vi "HEWH Stand Overide.vi"() -> ()   [LabVIEW 2009]
uses:
  EquipReferences.ctl
  HEWH Tank Indicator.ctl
  Intellifaucet/Intellfaucet Mode.ctl
  PowerElements.ctl
  ChannelSettings.ctl
  <vilib>/Utility/file.llb/Write To Spreadsheet File (string).vi
panel:
  in  "Equipment":T1={"COM Port"="COM3", "MW100"="MW100", "AG34970"="A-34972A", "WT500"="WT500"}
  in  "Flow Calculation":bool
  out "Iteration":i32
  out "MW100":refnum<visa-resource-name>
  out "Local?":bool
  in  "Help":bool
  in  "VALVE OUT":enum8{"CLOSE", "OPEN"}(ring)
  in  "DRAIN VALVE":enum8{"OPEN", "CLOSE"}(ring)
  in  "INPUT VALVE":enum8{"OPEN", "CLOSE"}(ring)
  out "Error Out":errorcluster
  out "Ready":bool=TRUE
  in  "Stop Test":bool
  in  "HEWH Power":bool
  in  "Semiphore":T2
  in  "IF Stop":bool
  in  "IF Start":bool
  in  "IFaucet Driver":bool
  in  "Percent Flow":dbl(slide)=100.0 scale=0.0..100.0
  in  "Temperature(F)":dbl(slide)=58.0 scale=40.0..120.0
  in  "Mode":T3
  in  "Error In":errorcluster
  in  "Agilent?":bool=TRUE
  in  "No Serial Port Delay(mS, 250 mS increments)":u32=10000
  out "POWER":T4
  in  "Serial Port Available?":bool=TRUE
  in  "Write To File":bool
  in  "file path (dialog if empty)":path=path "C:/Data/data.csv"
  out "GatherDataCount":i32
  out "Output Data":string[][](array[string])
  out "Tank Display":T5 {"TC6" format="%.2g"; "TIN" format="%.2g"; "TOUT" format="%.2g"; "Mean" format="%.2f"; "Std Dev" format="%.2f"; "TC5" format="%.2g"; "TC4" format="%.2g"; "TC3" format="%.2g"; "TC2" format="%.2g"; "TC1" format="%.2g"}
  in  "Gather Data":bool
  in  "Test Condition":T6(ring)=enum."SRK500,Station1,5GPM FR"
  out "Dispensed":dbl
  out "ToutMin":dbl
  out "ToutMax":dbl
  in  "Gallon Target":dbl=10.72
  in  "GPM Target":dbl=3.0
  in  "Dispense":bool
  out "LBS":dbl
  in  "Reset Computations":bool
  out "Gallons":dbl
  out "BUG array":string[](array[string])
  out "Flow Chart":dbl(graph)
  out "Flow":dbl
  in  "Read Flow":bool
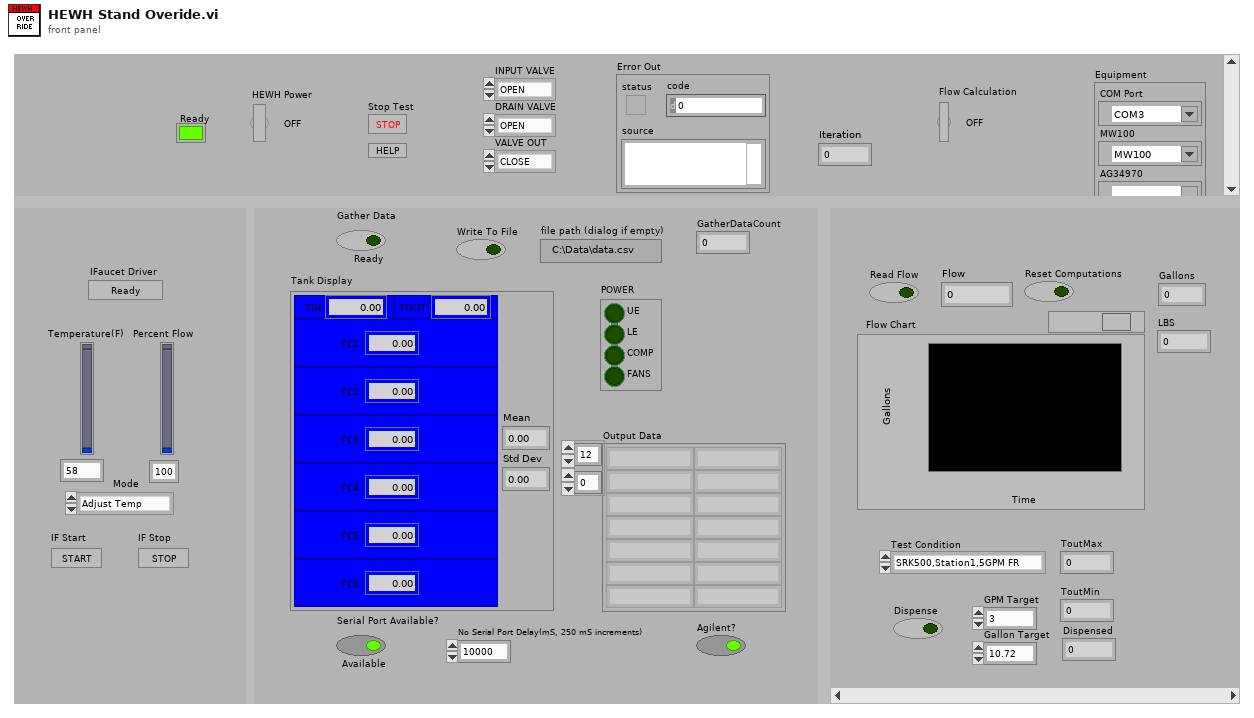
[diagram p1: front panel]
types:
  T1 = typedef "EquipReferences.ctl" = cluster{"COM Port":refnum<visa-resource-name>, "MW100":refnum<visa-resource-name>, "AG34970":refnum<visa-resource-name>, "WT500":refnum<visa-resource-name>}
  T2 = typedef "Semaphore RefNum" = refnum<k1>
  T3 = typedef "Intellfaucet Mode.ctl" = enum16{"Adjust Temp", "Adjust Flow", "Start Flow", "Stop Flow"}
  T4 = typedef "PowerElements.ctl" = cluster{"UE":bool, "LE":bool, "COMP":bool, "FANS":bool}
  T5 = typedef "HEWH Tank Indicator.ctl" = cluster{"TC1-D":bool, "TC2-D":bool, "TC3-D":bool, "TC4-D":bool, "TC5-D":bool, "RTD_IN":bool, "RTDOUT":bool, "TC1":dbl, "TC2":dbl, "TC3":dbl, "TC4":dbl, "TC5":dbl, "TIN":dbl, "TOUT":dbl, "Std Dev":dbl, "Mean":dbl, "TC6-D":bool, "TC6":dbl}
  T6 = enum16{"DRK500,Station1", "DRK375,Lab", "SRK500,Station1,5GPM FR", "DRK500,Station1,downspout"}
  T7 = typedef "ChannelSettings.ctl" = u32
  T8 = enum16{"Computation Start", "Computation stop", "Reset Computation", "Clear Computation"}
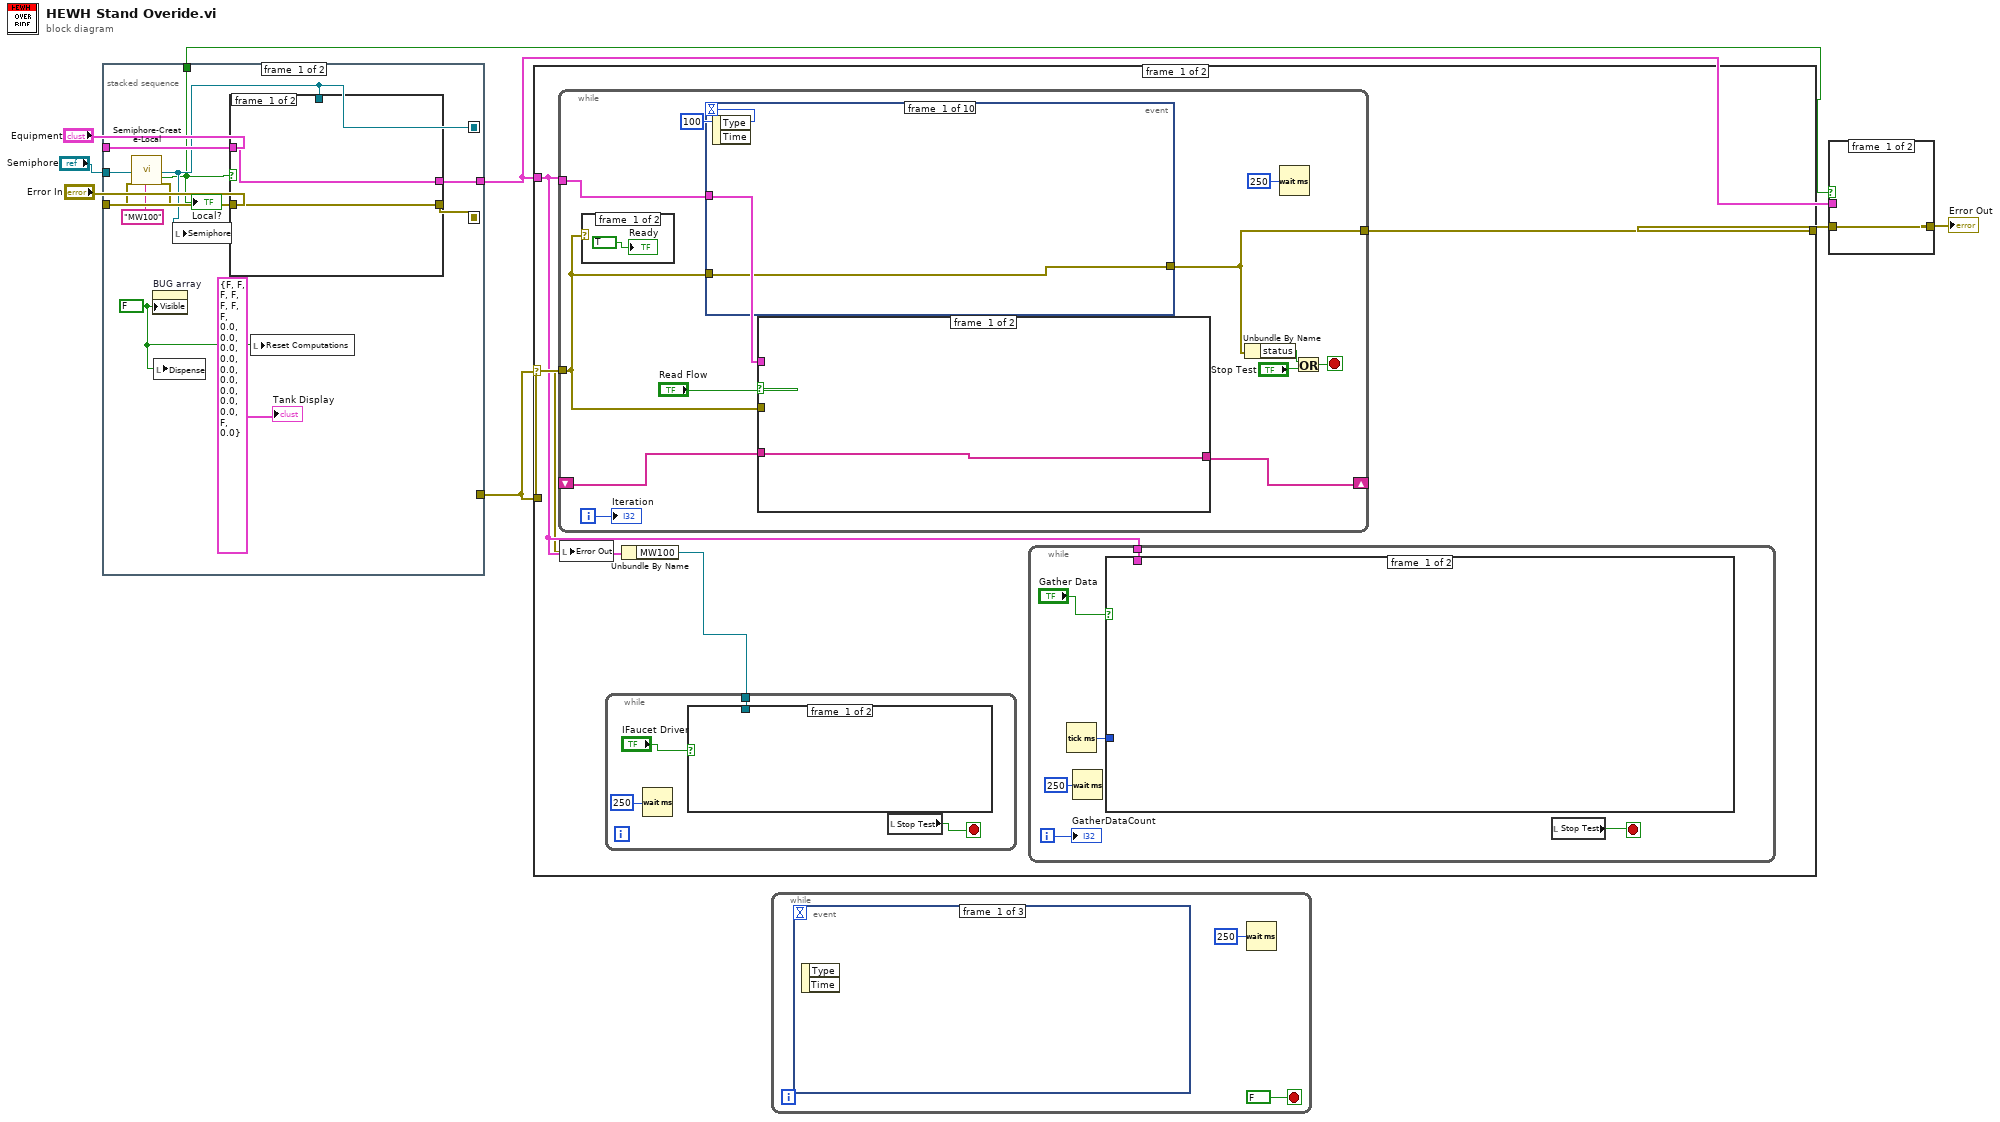
[diagram p0: block diagram]
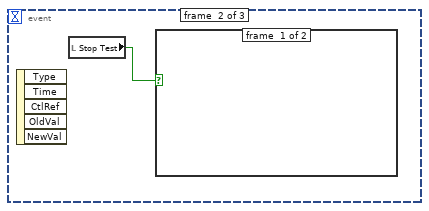
[diagram p2: hidden frame]
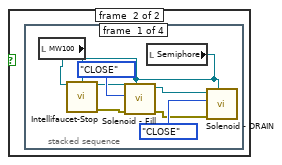
[diagram p3: hidden frame]
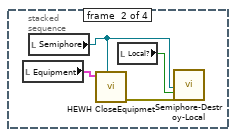
[diagram p4: hidden frame]
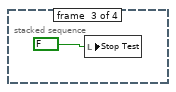
[diagram p5: hidden frame]
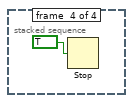
[diagram p6: hidden frame]
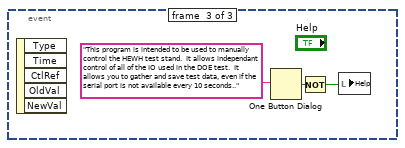
[diagram p7: hidden frame]
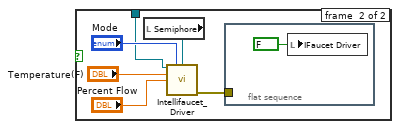
[diagram p8: hidden frame]
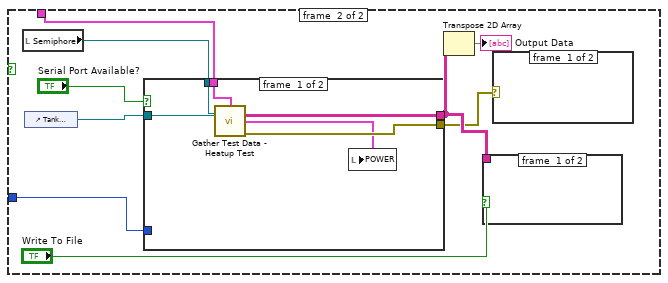
[diagram p9: hidden frame]
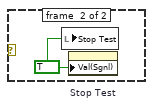
[diagram p10: hidden frame]
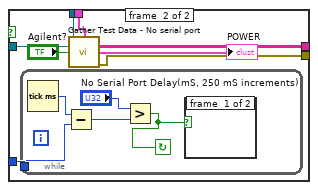
[diagram p11: hidden frame]
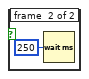
[diagram p12: hidden frame]
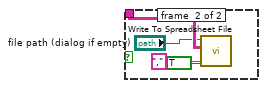
[diagram p13: hidden frame]
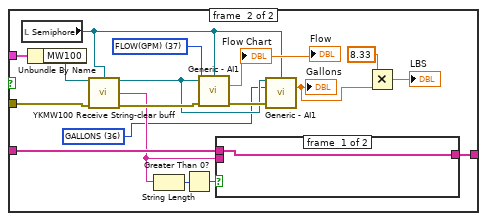
[diagram p14: hidden frame]
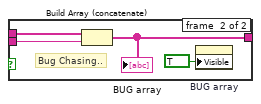
[diagram p15: hidden frame]
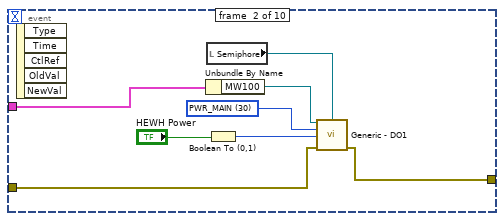
[diagram p17: hidden frame]
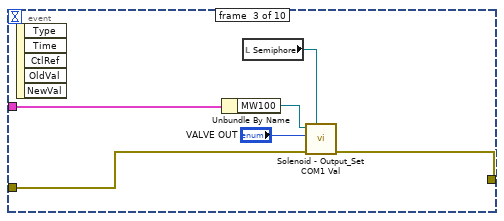
[diagram p18: hidden frame]
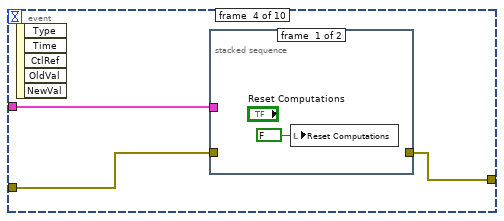
[diagram p19: hidden frame]
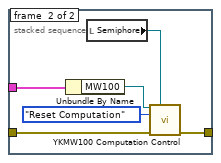
[diagram p20: hidden frame]
diagram:
  n1 = stacked-sequence {
    seq-local: [w17 _] -> [_ w45]
    seq-local: [w12 _] -> [_ w31]
    tunnel: "Error In" -> [w16 _]
    tunnel: "Equipment" -> [w19 w46]
    tunnel: [w18 _] -> w4
    tunnel: [_ w41] -> w3
    tunnel: [w11 _] -> w2
    tunnel: "Semiphore" -> [w14 _]
    frame #0 {
      w9 = FALSE ("Visible")
      n2 = call "Semiphore-Create-Local.vi"("Semiphore"=w14, "error in (no error)"=w16, "name (unnamed)"="MW100") -> ("semaphore"=w12:T2, "Local?"=w11:bool, "error out"=w15:errorcluster)  [unwired: 14 in]
      "Local?" <- w11
      n3 = property on="BUG array" class="Arr (strict)"("Visible"=w9) -> ()  [unwired: 2 in, 2 out]
      n4 = local write "Dispense"(w9) -> ()
      n5 = local write "Semiphore"(w12) -> ()
      n6 = case shown="True" w11 {
        tunnel: w15 -> [w21 w28]
        tunnel: [w21 w27] -> w17
        tunnel: w19 -> [w20 w26]
        tunnel: [w20 w23] -> w18
        tunnel: w12 -> [_ w24]
        frame #0 {
        }
        frame #1 {
          n7 = call "HEWH InitializeEquipmet.vi"("Semiphore"=w24, "Error In"=w28, "Equipment"=w26) -> ("Error Out"=w27:errorcluster, "Equipment Out"=w23:T1)  [unwired: 7 in]
          n8 = local write "Ready"(FALSE ("Ready")) -> ()
          n9 = Unbundle(w23) -> ("MW100"=→"MW100":refnum<visa-resource-name>)  [unwired: 3 out]
        }
      }
      n10 = local write "Reset Computations"(w9) -> ()
      "Tank Display" <- T5 {"TC1-D"=FALSE, "TC2-D"=FALSE, "TC3-D"=FALSE, "TC4-D"=FALSE, "TC5-D"=FALSE, "RTD_IN"=FALSE, "RTDOUT"=FALSE, "TC1"=0.0, "TC2"=0.0, "TC3"=0.0, "TC4"=0.0, "TC5"=0.0, "TIN"=0.0, "TOUT"=0.0, "Std Dev"=0.0, "Mean"=0.0, "TC6-D"=FALSE, "TC6"=0.0} ("Tank Display")
    }
    frame #1 {
      w32 = FALSE ("Stop Test")
      w36 = T7 30 items=["4-20_OUT", "Pres_HI1", "Pres_HI2", "Pres_LOW", "Pres_PIN", "HEATER_TOP", "HEATER_BOT", "T_Shell", "FLOWMETER", "WATT_SENSE", "WH_TICK", "Tc_1", "Tc_2", "Tc_3", "Tc_4", "Tc_5", "Tc_6", "Tc_down", "T_Shell_2", "T_Shell_3", "T_Shell_4", "RTD_IN", "RTD_OUT", "RTD_AMB", "INTF_TEMPFLO", "INTF_READY", "INTF_START", "INTF_STOP", "DRM_LOW", "DRM_HIGH", "PWR_MAIN", "VLV_DUMP", "VLV_OUT", "VLV_IN", "WATT_HOURS", "FLOW(SAMPLE)", "GALLONS", "FLOW(GPM)"] ("Channel_Enum")
      w37 = T7 33 items=["4-20_OUT", "Pres_HI1", "Pres_HI2", "Pres_LOW", "Pres_PIN", "HEATER_TOP", "HEATER_BOT", "T_Shell", "FLOWMETER", "WATT_SENSE", "WH_TICK", "Tc_1", "Tc_2", "Tc_3", "Tc_4", "Tc_5", "Tc_6", "Tc_down", "T_Shell_2", "T_Shell_3", "T_Shell_4", "RTD_IN", "RTD_OUT", "RTD_AMB", "INTF_TEMPFLO", "INTF_READY", "INTF_START", "INTF_STOP", "DRM_LOW", "DRM_HIGH", "PWR_MAIN", "VLV_DUMP", "VLV_OUT", "VLV_IN", "WATT_HOURS", "FLOW(SAMPLE)", "GALLONS", "FLOW(GPM)"] ("Channel_Enum")
      w38 = T7 32 items=["4-20_OUT", "Pres_HI1", "Pres_HI2", "Pres_LOW", "Pres_PIN", "HEATER_TOP", "HEATER_BOT", "T_Shell", "FLOWMETER", "WATT_SENSE", "WH_TICK", "Tc_1", "Tc_2", "Tc_3", "Tc_4", "Tc_5", "Tc_6", "Tc_down", "T_Shell_2", "T_Shell_3", "T_Shell_4", "RTD_IN", "RTD_OUT", "RTD_AMB", "INTF_TEMPFLO", "INTF_READY", "INTF_START", "INTF_STOP", "DRM_LOW", "DRM_HIGH", "PWR_MAIN", "VLV_DUMP", "VLV_OUT", "VLV_IN", "WATT_HOURS", "FLOW(SAMPLE)", "GALLONS", "FLOW(GPM)"] ("Channel_Enum")
      w40 = T7 31 items=["4-20_OUT", "Pres_HI1", "Pres_HI2", "Pres_LOW", "Pres_PIN", "HEATER_TOP", "HEATER_BOT", "T_Shell", "FLOWMETER", "WATT_SENSE", "WH_TICK", "Tc_1", "Tc_2", "Tc_3", "Tc_4", "Tc_5", "Tc_6", "Tc_down", "T_Shell_2", "T_Shell_3", "T_Shell_4", "RTD_IN", "RTD_OUT", "RTD_AMB", "INTF_TEMPFLO", "INTF_READY", "INTF_START", "INTF_STOP", "DRM_LOW", "DRM_HIGH", "PWR_MAIN", "VLV_DUMP", "VLV_OUT", "VLV_IN", "WATT_HOURS", "FLOW(SAMPLE)", "GALLONS", "FLOW(GPM)"] ("Channel_Enum")
      n11 = Unbundle By Name(w46) -> ("MW100"=w39:refnum<visa-resource-name>)
      n12 = local write "Stop Test"(w32) -> ()
      n13 = local write "Ready"(w32) -> ()
      n14 = local write "IFaucet Driver"(w32) -> ()
      n15 = call "YKMW100 VF0 Relay Status.vi"("VISA session"=w39, "Semiphore"=w31, "Channel_Enum"=w36, "error in (no error)"=w45) -> ("x = y?"=w29:bool, "error out"=w44:errorcluster)  [unwired: 9 in, 1 out]
      n16 = call "YKMW100 VF0 Relay Status.vi"("VISA session"=w39, "Semiphore"=w31, "Channel_Enum"=w37, "error in (no error)"=w44) -> ("x = y?"=w35:bool, "error out"=w43:errorcluster)  [unwired: 9 in, 1 out]
      n17 = call "YKMW100 VF0 Relay Status.vi"("VISA session"=w39, "Semiphore"=w31, "Channel_Enum"=w38, "error in (no error)"=w43) -> ("x = y?"=w34:bool, "error out"=w42:errorcluster)  [unwired: 9 in, 1 out]
      n18 = call "YKMW100 VF0 Relay Status.vi"("VISA session"=w39, "Semiphore"=w31, "Channel_Enum"=w40, "error in (no error)"=w42) -> ("x = y?"=w33:bool, "error out"=w41:errorcluster)  [unwired: 9 in, 1 out]
      n19 = Not(x=w29) -> (.not. x?=w30:bool)
      n20 = case shown="False" w35 {
        frame #0 {
          n21 = local write "INPUT VALVE"(enum8{"OPEN", "CLOSE"}."CLOSE" ("INPUT VALVE")) -> ()
        }
        frame #1 {
          n22 = local write "INPUT VALVE"(enum8{"OPEN", "CLOSE"}."OPEN" ("INPUT VALVE")) -> ()
        }
      }
      n23 = case shown="False" w33 {
        frame #0 {
          n24 = local write "DRAIN VALVE"(enum8{"OPEN", "CLOSE"}."OPEN" ("DRAIN VALVE")) -> ()
        }
        frame #1 {
          n25 = local write "DRAIN VALVE"(enum8{"OPEN", "CLOSE"}."CLOSE" ("DRAIN VALVE")) -> ()
        }
      }
      n26 = case shown="False" w34 {
        frame #0 {
          n27 = local write "VALVE OUT"(enum8{"CLOSE", "OPEN"}."CLOSE" ("VALVE OUT")) -> ()
        }
        frame #1 {
          n28 = local write "VALVE OUT"(enum8{"CLOSE", "OPEN"}."OPEN" ("VALVE OUT")) -> ()
        }
      }
      n29 = local write "HEWH Power"(w30) -> ()
    }
  }
  n30 = case shown="No Error" w3 {
    selector: w3 -> [w53 _]
    tunnel: [w57 w216] -> w7
    tunnel: w3 -> [w56 w216]
    tunnel: w4 -> [w55 _]
    frame #0 {
      n31 = while {
        tunnel: w56 -> [w111]
        tunnel: [w116] -> w57
        shift-right: [w113] -> _
        shift-left: _ -> [w112]
        tunnel: w55 -> [w110]
        i -> [w114]
        stop <- w117 stop-if-true
        n32 = case shown="No Error" w111 {
          frame #0 {
            "Ready" <- TRUE
          }
          frame #1 {
          }
        }
        n33 = event shown="[7] \"IF Start\": Value Change" {
          selector: _ -> [_ _ _ _ _ _ _ _ _ _]
          dyn-events: _ -> [_ _ _ _ _ _ _ _ _ _]
          timeout: 100 -> [_ _ _ _ _ _ _ _ _ _]
          tunnel: w111 -> [w146 w152 w156 w162 w181 w186 w190 w196 w203 w211]
          tunnel: [w146 w148 w157 w161 w173 w185 w189 w195 w202 w210] -> w116
          tunnel: w110 -> [_ w151 w160 w163 w180 w188 w194 w199 w205 w214]
          event #0 {
            n34 = event-data() -> ()  [unwired: 1 in, 2 out]
          }
          event #1 {
            w150 = T7 30 items=["4-20_OUT", "Pres_HI1", "Pres_HI2", "Pres_LOW", "Pres_PIN", "HEATER_TOP", "HEATER_BOT", "T_Shell", "FLOWMETER", "WATT_SENSE", "WH_TICK", "Tc_1", "Tc_2", "Tc_3", "Tc_4", "Tc_5", "Tc_6", "Tc_down", "T_Shell_2", "T_Shell_3", "T_Shell_4", "RTD_IN", "RTD_OUT", "RTD_AMB", "INTF_TEMPFLO", "INTF_READY", "INTF_START", "INTF_STOP", "DRM_LOW", "DRM_HIGH", "PWR_MAIN", "VLV_DUMP", "VLV_OUT", "VLV_IN", "WATT_HOURS", "FLOW(SAMPLE)", "GALLONS", "FLOW(GPM)"] ("Channel_Enum")
            n35 = event-data() -> ()  [unwired: 1 in, 5 out]
            n36 = Unbundle By Name(w151) -> ("MW100"=w153:refnum<visa-resource-name>)
            n37 = local read "Semiphore"() -> (w149:T2)
            n38 = Boolean To (0,1)(Boolean="HEWH Power") -> (0, 1=w154:i16)
            n39 = call "Generic - DO1.vi"("VISA session"=w153, "Semiphore"=w149, "Channel_Enum"=w150, "Relay Status (0:CLOSED)"=w154, "Error In"=w152) -> ("error out"=w148:errorcluster)  [unwired: 9 in, 1 out]
          }
          event #2 {
            n40 = event-data() -> ()  [unwired: 1 in, 5 out]
            n41 = Unbundle By Name(w160) -> ("MW100"=w159:refnum<visa-resource-name>)
            n42 = local read "Semiphore"() -> (w158:T2)
            n43 = call "Solenoid - Output_Set COM1 Val.vi"("Semiphore"=w158, "Error In"=w156, "OPEN CLOSE"="VALVE OUT", "VISA session"=w159) -> ("Error Out"=w157:errorcluster)  [unwired: 6 in, 1 out]
          }
          event #3 {
            n44 = event-data() -> ()  [unwired: 1 in, 5 out]
            n45 = stacked-sequence {
              tunnel: w163 -> [_ w170]
              tunnel: w162 -> [_ w167]
              tunnel: [_ w165] -> w161
              frame #0 {
                n46 = local write "Reset Computations"(FALSE ("Reset Computations")) -> ()
              }
              frame #1 {
                n47 = Unbundle By Name(w170) -> ("MW100"=w169:refnum<visa-resource-name>)
                n48 = local read "Semiphore"() -> (w168:T2)
                n49 = call "YKMW100 Computation Control.vi"("VISA session"=w169, "Semiphore"=w168, "Mode"=T8."Reset Computation", "error in (no error)"=w167) -> ("error out"=w165:errorcluster)  [unwired: 10 in, 1 out]
              }
            }
          }
          event #4 {
            n50 = event-data() -> ()  [unwired: 1 in, 5 out]
            n51 = control-ref of="Flow Chart"() -> (w172:refnum<vi>)
            n52 = local read "Semiphore"() -> (w179:T2)
            n53 = call "Dispense X Gallon at Y Flowrate.vi"("Gallon Target"="Gallon Target", "Equipment"=w180, "Semiphore"=w179, "GPM Target"="GPM Target", "Test Condition"="Test Condition", "Error In"=w181, "Ctl Refnum"=w172) -> ("M*(Gallons)"=→"Dispensed":dbl, "ToutMax"=→"ToutMax":dbl, "ToutMin"=→"ToutMin":dbl, "Error Out"=w173:errorcluster)  [unwired: 3 in, 2 out]
            n54 = flat-sequence {
              tunnel: w173 -> [_]
              frame #0 {
                n55 = local write "Dispense"(FALSE ("IF Start")) -> ()
              }
            }
          }
          event #5 {
            n56 = event-data() -> ()  [unwired: 1 in, 5 out]
            n57 = Unbundle By Name(w188) -> ("MW100"=w183:refnum<visa-resource-name>)
            n58 = local read "Semiphore"() -> (w184:T2)
            n59 = call "Solenoid - Fill.vi"("Semiphore"=w184, "Error In"=w186, "VALVE OPEN CLOSE"="INPUT VALVE", "VISA session"=w183) -> ("Error Out"=w185:errorcluster)  [unwired: 6 in, 1 out]
          }
          event #6 {
            n60 = event-data() -> ()  [unwired: 1 in, 5 out]
            n61 = Unbundle By Name(w194) -> ("MW100"=w192:refnum<visa-resource-name>)
            n62 = local read "Semiphore"() -> (w193:T2)
            n63 = call "Solenoid - DRAIN.vi"("Semiphore"=w193, "Error In"=w190, "VALVE OPEN CLOSE"="DRAIN VALVE", "VISA session"=w192) -> ("Error Out"=w189:errorcluster)  [unwired: 6 in, 1 out]
          }
          event #7 {
            n64 = event-data() -> ()  [unwired: 1 in, 5 out]
            n65 = Unbundle By Name(w199) -> ("MW100"=w197:refnum<visa-resource-name>)
            n66 = local read "Semiphore"() -> (w198:T2)
            n67 = call "Intellifaucet-Start.vi"("Semiphore"=w198, "Error In"=w196, "VISA session"=w197) -> ("Error Out"=w195:errorcluster)  [unwired: 7 in, 1 out]
            n68 = flat-sequence {
              tunnel: w195 -> [_]
              frame #0 {
                n69 = local write "IF Start"(FALSE ("IF Start")) -> ()
              }
            }
          }
          event #8 {
            n70 = event-data() -> ()  [unwired: 1 in, 5 out]
            n71 = Unbundle By Name(w205) -> ("MW100"=w204:refnum<visa-resource-name>)
            n72 = local read "Semiphore"() -> (w201:T2)
            n73 = Select(t="001" ("Value"), s="Flow Calculation", f="000" ("Value")) -> (s? t:f=w206:string)
            n74 = call "YKMW100 Write Com Register.vi"("VISA session"=w204, "Semiphore"=w201, "Value"=w206, "error in (no error)"=w203) -> ("error out"=w202:errorcluster)  [unwired: 10 in, 1 out]
          }
          event #9 {
            n75 = event-data() -> ()  [unwired: 1 in, 5 out]
            n76 = Unbundle By Name(w214) -> ("MW100"=w212:refnum<visa-resource-name>)
            n77 = local read "Semiphore"() -> (w213:T2)
            n78 = call "Intellifaucet-Stop.vi"("VISA session"=w212, "Semiphore"=w213, "Error In"=w211) -> ("Error Out"=w210:errorcluster)  [unwired: 11 in, 1 out]
            n79 = flat-sequence {
              tunnel: w210 -> [_]
              frame #0 {
                n80 = local write "IF Stop"(FALSE ("IF Start")) -> ()
              }
            }
          }
        }
        n81 = case shown="True" "Read Flow" {
          tunnel: w110 -> [_ w139]
          tunnel: w111 -> [_ w137]
          tunnel: [w121 w135] -> w113
          tunnel: w112 -> [w121 w134]
          frame #0 {
          }
          frame #1 {
            w125 = T7 36 items=["4-20_OUT", "Pres_HI1", "Pres_HI2", "Pres_LOW", "Pres_PIN", "HEATER_TOP", "HEATER_BOT", "T_Shell", "FLOWMETER", "WATT_SENSE", "WH_TICK", "Tc_1", "Tc_2", "Tc_3", "Tc_4", "Tc_5", "Tc_6", "Tc_down", "T_Shell_2", "T_Shell_3", "T_Shell_4", "RTD_IN", "RTD_OUT", "RTD_AMB", "INTF_TEMPFLO", "INTF_READY", "INTF_START", "INTF_STOP", "DRM_LOW", "DRM_HIGH", "PWR_MAIN", "VLV_DUMP", "VLV_OUT", "VLV_IN", "WATT_HOURS", "FLOW(SAMPLE)", "GALLONS", "FLOW(GPM)"] ("Channel_Enum")
            w130 = T7 37 items=["4-20_OUT", "Pres_HI1", "Pres_HI2", "Pres_LOW", "Pres_PIN", "HEATER_TOP", "HEATER_BOT", "T_Shell", "FLOWMETER", "WATT_SENSE", "WH_TICK", "Tc_1", "Tc_2", "Tc_3", "Tc_4", "Tc_5", "Tc_6", "Tc_down", "T_Shell_2", "T_Shell_3", "T_Shell_4", "RTD_IN", "RTD_OUT", "RTD_AMB", "INTF_TEMPFLO", "INTF_READY", "INTF_START", "INTF_STOP", "DRM_LOW", "DRM_HIGH", "PWR_MAIN", "VLV_DUMP", "VLV_OUT", "VLV_IN", "WATT_HOURS", "FLOW(SAMPLE)", "GALLONS", "FLOW(GPM)"] ("Channel_Enum")
            n82 = local read "Semiphore"() -> (w126:T2)
            n83 = Unbundle By Name(w139) -> ("MW100"=w138:refnum<visa-resource-name>)
            n84 = call "YKMW100 Receive String-clear buff.vi"("VISA session"=w138, "Semiphore"=w126, "error in (no error)"=w137) -> ("dup VISA session"=w127:refnum<visa-resource-name>, "Read Buffer"=w133:string, "error out"=w136:errorcluster)  [unwired: 10 in]
            n85 = String Length(string=w133) -> (length=w132:i32)
            n86 = Greater Than 0?(x=w132) -> (x > 0?=w131:bool)
            n87 = call "Generic - AI1.vi"("MW100"=w127, "Semiphore"=w126, "Channel_Enum"=w130, "Error In"=w136) -> ("Value"=→"Flow" →"Flow Chart":dbl, "Error Out"=w128:errorcluster)  [unwired: 9 in, 1 out]
            n88 = case shown="True" w131 {
              tunnel: w133 -> [_ w144]
              tunnel: [w140 w142] -> w135
              tunnel: w134 -> [w140 w143]
              frame #0 {
              }
              frame #1 {
                # "Bug Chasing.."
                n89 = Build Array (concatenate)(w143, w144) -> (w142:string[])
                "BUG array" <- w142
                n90 = property on="BUG array" class="Arr (strict)"("Visible"=TRUE) -> ()  [unwired: 2 in, 2 out]
              }
            }
            n91 = call "Generic - AI1.vi"("MW100"=w127, "Semiphore"=w126, "Channel_Enum"=w125, "Error In"=w128) -> ("Value"=w124:dbl)  [unwired: 9 in, 2 out]
            "Gallons" <- w124
            n92 = Multiply(x=8.33, y=w124) -> (x*y=→"LBS":dbl)
          }
        }
        n93 = Unbundle By Name(w116) -> ("status"=w118:bool)
        n94 = Wait (ms)(milliseconds to wait=u32 250) -> ()  [unwired: 1 out]
        n95 = Or(x=w118, y="Stop Test") -> (x .or. y?=w117:bool)
        "Iteration" <- w114
      }
      n96 = local write "Error Out"(w53) -> ()
      n97 = Unbundle By Name(w55) -> ("MW100"=w54:refnum<visa-resource-name>)
      n98 = while {
        tunnel: w54 -> [w59]
        stop <- w60 stop-if-true
        n99 = Wait (ms)(milliseconds to wait=u32 250) -> ()  [unwired: 1 out]
        n100 = case shown="True" "IFaucet Driver" {
          tunnel: w59 -> [_ w63]
          frame #0 {
          }
          frame #1 {
            n101 = local read "Semiphore"() -> (w67:T2)
            n102 = call "Intellifaucet_Driver.vi"("VISA session"=w63, "Mode"="Mode", "Semiphore"=w67, "Temperature(F)"="Temperature(F)", "Percent Flow"="Percent Flow") -> ("Error Out"=w62:errorcluster)  [unwired: 9 in, 1 out]
            n103 = flat-sequence {
              tunnel: w62 -> [_]
              frame #0 {
                n104 = local write "IFaucet Driver"(FALSE ("IFaucet Driver")) -> ()
              }
            }
          }
        }
        n105 = local read "Stop Test"() -> (w60:bool)
      }
      n106 = while {
        tunnel: w55 -> [w72]
        i -> [w71]
        stop <- w73 stop-if-true
        n107 = Tick Count (ms)() -> (millisecond timer value=w69:u32)
        n108 = Wait (ms)(milliseconds to wait=u32 250) -> ()  [unwired: 1 out]
        n109 = case shown="True" "Gather Data" {
          tunnel: w72 -> [_ w80]
          tunnel: w69 -> [_ w75]
          frame #0 {
          }
          frame #1 {
            n110 = local read "Semiphore"() -> (w82:T2)
            n111 = control-ref of="Tank Display"() -> (w81:refnum<vi>)
            n112 = case shown="False" "Serial Port Available?" {
              tunnel: w82 -> [w90 w98]
              tunnel: w81 -> [w89 w97]
              tunnel: w80 -> [w88 w96]
              tunnel: [w87 w95] -> w79
              tunnel: [w86 w94] -> w76
              tunnel: w75 -> [_ w92]
              frame #0 {
                n113 = call "Gather Test Data - Heatup Test.vi"("Semiphore"=w90, "Equipment"=w88, "Tank Display Ref"=w89) -> ("Output Data"=w87:string[][], "POWER"=w85:T4, "error out"=w86:errorcluster)  [unwired: 8 in, 2 out]
                n114 = local write "POWER"(w85) -> ()
              }
              frame #1 {
                n115 = while {
                  tunnel: w92 -> [w102]
                  stop <- w99 continue-if-true
                  n116 = Tick Count (ms)() -> (millisecond timer value=w103:u32)
                  n117 = Subtract(x=w103, y=w102) -> (x-y=w100:u32)
                  n118 = Greater?(x="No Serial Port Delay(mS, 250 mS increments)", y=w100) -> (0:w99:bool)
                  n119 = case shown="True" w99 {
                    frame #0 {
                    }
                    frame #1 {
                      n120 = Wait (ms)(milliseconds to wait=u32 250) -> ()  [unwired: 1 out]
                    }
                  }
                }
                n121 = call "Gather Test Data - No serial port.vi"("Semiphore"=w98, "Equipment"=w96, "Tank Display Ref"=w97, "Agilent?"="Agilent?") -> ("Output Data"=w95:string[][], "POWER"=→"POWER":T4, "error out"=w94:errorcluster)  [unwired: 7 in, 2 out]
              }
            }
            n122 = Transpose 2D Array(2D array=w79) -> (transposed array=→"Output Data":string[][])
            n123 = case shown="True" "Write To File" {
              tunnel: w79 -> [_ w108]
              frame #0 {
              }
              frame #1 {
                n124 = call-poly <vilib>:"Write To Spreadsheet File.vi"("delimiter (\\t)"="," ("delimiter (\\t)"), "append to file? (new file:F)"=TRUE, "2D data"=w108, "file path (dialog if empty)"="file path (dialog if empty)") -> ()  [unwired: 4 in, 1 out]
              }
            }
            n125 = case shown="Error" w76 {
              frame #0 {
              }
              frame #1 {
                w84 = TRUE ("Value (Signaling)")
                n126 = local write "Stop Test"(w84) -> ()
                n127 = property on="Stop Test" class="Bool (strict)"("Val(Sgnl)"=w84) -> ()  [unwired: 2 in, 2 out]
              }
            }
          }
        }
        n128 = local read "Stop Test"() -> (w73:bool)
        "GatherDataCount" <- w71
      }
    }
    frame #1 {
    }
  }
  n129 = while {
    stop <- FALSE stop-if-true
    n130 = event shown="[1] \"Stop Test\": Value Change" {
      selector: _ -> [_ _ _]
      dyn-events: _ -> [_ _ _]
      timeout: _ -> [_ _ _]
      event #0 {
        n131 = event-data() -> ()  [unwired: 1 in, 2 out]
      }
      event #1 {
        n132 = event-data() -> ()  [unwired: 1 in, 5 out]
        n133 = local read "Stop Test"() -> (w219:bool)
        n134 = case shown="True" w219 {
          frame #0 {
          }
          frame #1 {
            n135 = stacked-sequence {
              frame #0 {
                n136 = local read "MW100"() -> (w221:refnum<visa-resource-name>)
                n137 = local read "Semiphore"() -> (w220:T2)
                n138 = call "Intellifaucet-Stop.vi"("VISA session"=w221, "Semiphore"=w220) -> ("dup VISA session"=w223:refnum<visa-resource-name>, "Error Out"=w227:errorcluster)  [unwired: 12 in]
                n139 = call "Solenoid - Fill.vi"("Semiphore"=w220, "Error In"=w227, "VALVE OPEN CLOSE"=enum8{"OPEN", "CLOSE"}."CLOSE", "VISA session"=w223) -> ("Error Out"=w225:errorcluster, "dup VISA session"=w222:refnum<visa-resource-name>)  [unwired: 6 in]
                n140 = call "Solenoid - DRAIN.vi"("Semiphore"=w220, "Error In"=w225, "VALVE OPEN CLOSE"=enum8{"OPEN", "CLOSE"}."CLOSE", "VISA session"=w222) -> ()  [unwired: 6 in, 2 out]
              }
              frame #1 {
                n141 = local read "Equipment"() -> (w231:T1)
                n142 = local read "Semiphore"() -> (w230:T2)
                n143 = call "HEWH CloseEquipmet.vi"("Semiphore"=w230, "Equipment"=w231) -> ("Error Out"=w229:errorcluster)  [unwired: 9 in]
                n144 = local read "Local?"() -> (w228:bool)
                n145 = call "Semiphore-Destroy-Local.vi"("Semiphore"=w230, "Local?"=w228, "error in (no error)"=w229) -> ()  [unwired: 16 in, 1 out]
              }
              frame #2 {
                n146 = local write "Stop Test"(FALSE ("stop")) -> ()
              }
              frame #3 {
                n147 = Stop(stop? (T)=TRUE) -> ()
              }
            }
          }
        }
      }
      event #2 {
        n148 = event-data() -> ()  [unwired: 1 in, 5 out]
        n149 = One Button Dialog(message="This program is intended to be used to manually control the HEWH test stand.  It allows independant control of all of the IO used in the DOE test.  It allows you to gather and save test data, even if the serial port is not available every 10 seconds..") -> (true=w235:bool)  [unwired: 1 in]
        n150 = Not(x=w235) -> (.not. x?=w234:bool)
        n151 = local write "Help"(w234) -> ()
      }
    }
    n152 = Wait (ms)(milliseconds to wait=u32 250) -> ()  [unwired: 1 out]
  }
  n153 = case shown="True" w2 {
    tunnel: w7 -> [w237 w239]
    tunnel: [w237 w239] -> w5
    tunnel: w4 -> [_ w240]
    frame #0 {
    }
    frame #1 {
      n154 = local read "Semiphore"() -> (w238:T2)
      n155 = call "HEWH CloseEquipmet.vi"("Semiphore"=w238, "Equipment"=w240) -> ()  [unwired: 9 in, 1 out]
    }
  }
  "Error Out" <- w5
